vi "read_data_paths.vi"(8 "error in (no error)":errorcluster) -> (0 "error out":errorcluster, 3 "path [] out":path[](array[path]))   [LabVIEW 2015, in "lv-bin.lvlib" / "v1.lvlib"]
doc: "This vi allows you to get an array of all the data paths added using the add_data_path.vi"
uses:
  v1.lvlib
  lv-bin.lvlib
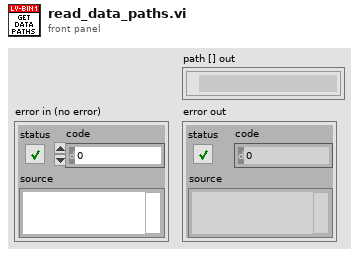
[diagram p1: front panel]
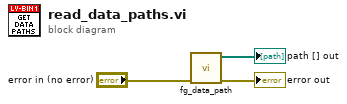
[diagram p0: block diagram]
diagram:
  n1 = call "fg_data_path.vi"("error in (no error)"="error in (no error)") -> ("error out"=→"error out":errorcluster, "path [] out"=→"path [] out":path[])  [unwired: 9 in]
